vi "Pre-Purge Start.vi"(8 "error in (no error)":errorcluster, 10 "Indicator states in":T2 {"Time Count" format="%.2g"}, 11 "Runtime statuses in":T1) -> (0 "error out":errorcluster, 2 "Indicator states out":T2 {"Time Count" format="%.2g"}, 3 "Runtime statuses out":T1)   [LabVIEW 2014]
doc: "Checks runtime statuses. If Pre-Purge is ready logs Start Pre-Purge event and alows next state: Pre-Purge"
uses:
  Controls/Boiler Status Indicators.ctl
  Controls/Boiler runtime status indicators.ctl
  Controls/Log file FGV action enum.ctl
  Controls/Log event enum.ctl
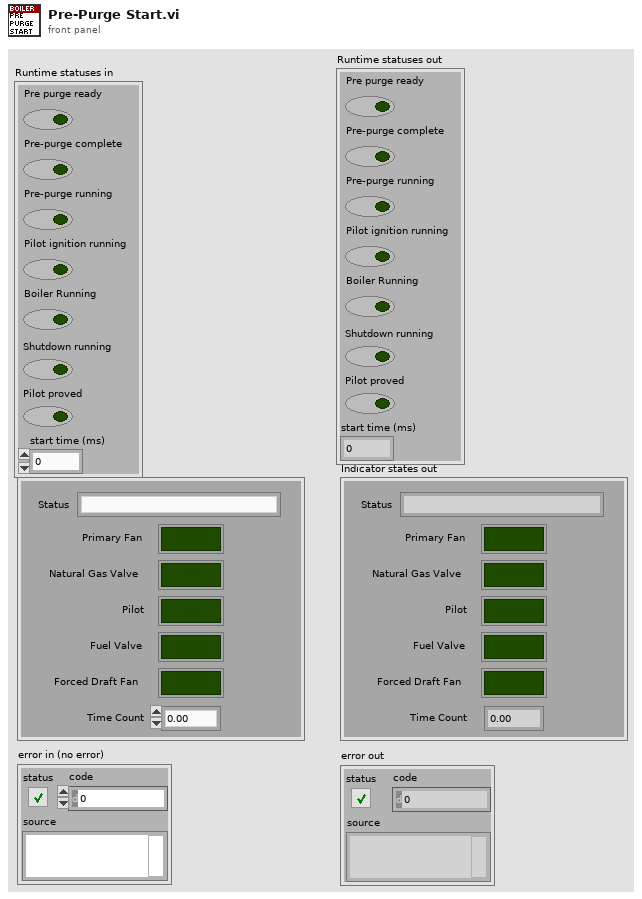
[diagram p1: front panel]
types:
  T1 = typedef "Boiler runtime status indicators.ctl" = cluster{"Pre purge ready":bool, "Pre-purge complete":bool, "Pre-purge running":bool, "Pilot ignition running":bool, "Boiler Running":bool, "Shutdown running":bool, "Pilot proved":bool, "start time (ms)":u32}
  T2 = typedef "Boiler Status Indicators.ctl" = cluster{"Status":string, "Primary Fan":bool, "Natural Gas Valve":bool, "Pilot":bool, "Fuel Valve":bool, "Forced Draft Fan":bool, "Time Count":dbl}
  T3 = typedef "Log event enum.ctl" = enum16{"Boiler Initialized", "Boiler Ready", "Start Pre-Purge", "Pre-Purge Complete", "Pilot ON", "Pilot proved", "Forced Draft Fan ON", "Boiler Running", "Start Shutdown Purge", "Shutdown Purge Complete"}
  T4 = typedef "Log file FGV action enum.ctl" = enum16{"open log file", "log event", "close log file"}
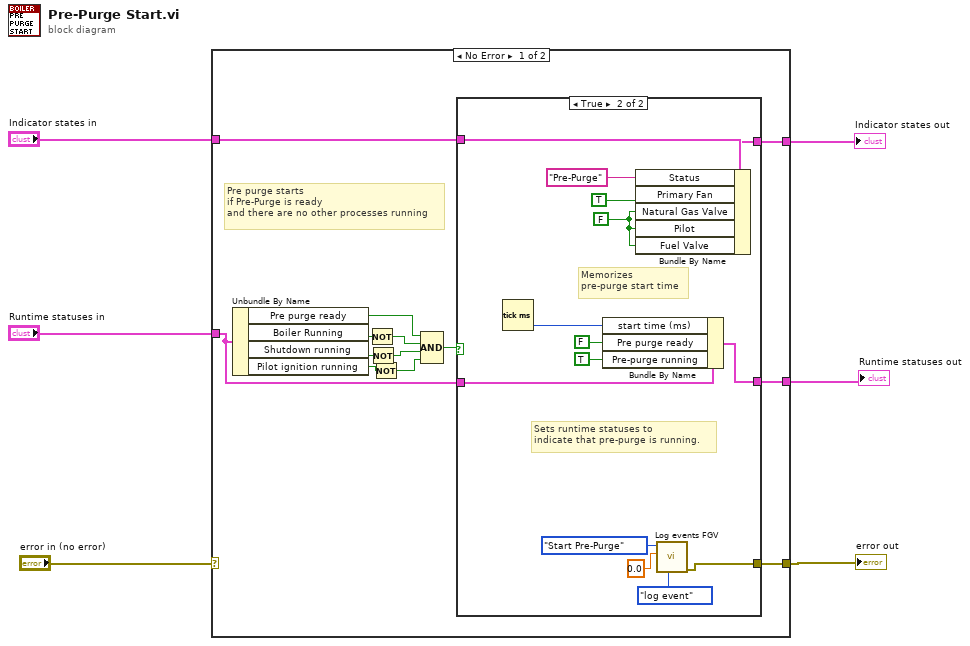
[diagram p0: block diagram]
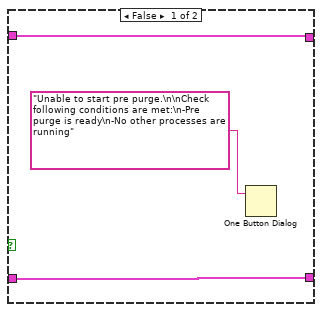
[diagram p2: hidden frame]
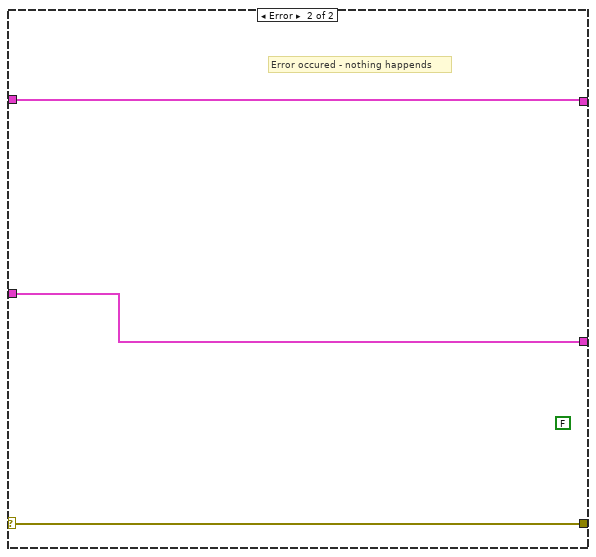
[diagram p3: hidden frame]
diagram:
  n1 = case shown="No Error" "error in (no error)" {
    selector: "error in (no error)" -> [_ w39]
    tunnel: [w7 w39] -> w5
    tunnel: "Runtime statuses in" -> [w12 w37]
    tunnel: "Indicator states in" -> [w14 w38]
    tunnel: [w13 w38] -> w2
    tunnel: [w11 w37] -> w1
    frame No Error {
      # "Pre purge starts\nif Pre-Purge is ready \nand there are no other processes running"
      n2 = Unbundle By Name(w12) -> ("Pre purge ready"=w10:bool, "Boiler Running"=w18:bool, "Shutdown running"=w19:bool, "Pilot ignition running"=w9:bool)
      n3 = Not(x=w18) -> (.not. x?=w17:bool)
      n4 = Not(x=w19) -> (.not. x?=w16:bool)
      n5 = Not(x=w9) -> (.not. x?=w8:bool)
      n6 = Compound Arithmetic op=AND(w10, w17, w16, w8) -> (w15:bool)
      n7 = case shown="True" w15 {
        tunnel: w14 -> [w22 w36]
        tunnel: [w22 w35] -> w13
        tunnel: w12 -> [w21 w33]
        tunnel: [w21 w32] -> w11
        tunnel: [_ w24] -> w7
        frame False {
          n8 = One Button Dialog(message="Unable to start pre purge.\n\nCheck following conditions are met:\n-Pre purge is ready\n-No other processes are running") -> ()  [unwired: 1 in, 1 out]
        }
        frame True {
          w27 = FALSE ("Natural Gas Valve")
          # "Memorizes\npre-purge start time"
          # "Sets runtime statuses to\nindicate that pre-purge is running."
          n9 = Tick Count (ms)() -> (millisecond timer value=w28:u32)
          n10 = Bundle By Name(cluster=w33, "start time (ms)"=w28, "Pre purge ready"=FALSE, "Pre-purge running"=TRUE ("Pre purge ready")) -> (w32:T1)
          n11 = Bundle By Name(cluster=w36, "Status"="Pre-Purge", "Primary Fan"=TRUE, "Natural Gas Valve"=w27, "Pilot"=w27, "Fuel Valve"=w27) -> (w35:T2)
          n12 = call "Log events FGV.vi"("action"=Log_file_FGV_action_enum."log event", "Event data"=0.0, "Log event"=Log_event_enum."Start Pre-Purge") -> ("error out"=w24:errorcluster)  [unwired: 8 in]
        }
      }
    }
    frame Error {
      (unwired) FALSE
      # "Error occured - nothing happends"
    }
  }
  "Indicator states out" <- w2
  "error out" <- w5
  "Runtime statuses out" <- w1
